vi "JsonEncoding.vi"() -> ()   [LabVIEW 2015]
uses:
  <vilib>/LVH/i3 JSON/JSON Generation/Create Value Files/Create Value - Array.vi
  <vilib>/LVH/i3 JSON/JSON Generation/Append to Array Files/Append to Array - Array.vi
  <vilib>/LVH/i3 JSON/i3-json.lvlib
panel:
  out "String":string
  out "Cluster":cluster{"Published Data 2":string[][]}={"Published Data 2"=[["Timestamp", "2016-04-14 13:40:56.035"], ["Wind Direction", "200.000000"], ["Wind Speed", "0.000000"], ["Air Temperature", "76.800000"], ["Internal Temperature", "76.800000"], ["Relative Humidity", "51.200000"], ["Air Pressure", "0.973400"], ["Rain Accumulation", "0.000000"], [" Rain Duration", "0.000000"], [" Rain Intensity", "0.000000"], ["Hail Duration", "0.000000"], [" Hail Intensity", "0.000000"], [" Supply Voltage", "5.100000"], [" Solar Irradiance", "4.296916"]]}
  in  "Published Data":string[][](array[string])
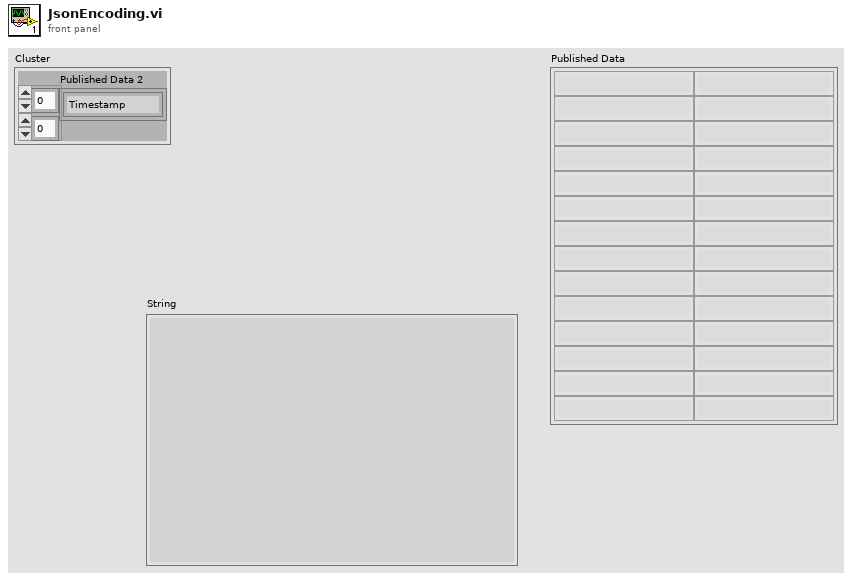
[diagram p1: front panel]
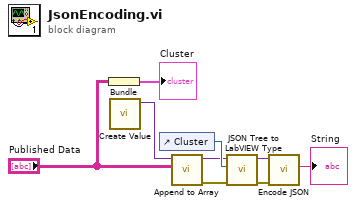
[diagram p0: block diagram]
diagram:
  n1 = Bundle("Published Data"="Published Data") -> (→"Cluster":cluster{"Published Data":string[][]})  [unwired: 1 in]
  n2 = call-poly <vilib>:"Create Value.vi"() -> ("JSON Tree"=w4:variant)  [unwired: 10 in, 1 out]
  n3 = control-ref of="Cluster"() -> (w9:refnum<vi>)
  n4 = call-poly <vilib>:"Append to Array.vi"("JSON Array"="Published Data", "JSON Tree in (JSON Array)"=w4) -> ("error out"=w3:errorcluster, "JSON Tree out (JSON Array)"=w2:variant)  [unwired: 8 in]
  n5 = call <vilib>:"JSON Tree to LabVIEW Type.vi"("error in (no error)"=w3, "Ctl Refnum"=w9, "JSON Tree In"=w2) -> ("error out"=w6:errorcluster, "JSON Tree Passthrough"=w7:variant)  [unwired: 7 in]
  n6 = call <vilib>:"Encode JSON.vi"("error in (no error)"=w6, "JSON Tree"=w7) -> ("String"=→"String":string)  [unwired: 4 in, 1 out]
